vi "Compare-Results.vi"(10 "FFT {X}":csg[](array[numeric]), 11 "Array in":csg[](array[numeric])) -> (2 "Numeric":i32, 3 "Boolean":bool)   [LabVIEW 2015]
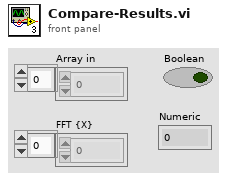
[diagram p1: front panel]
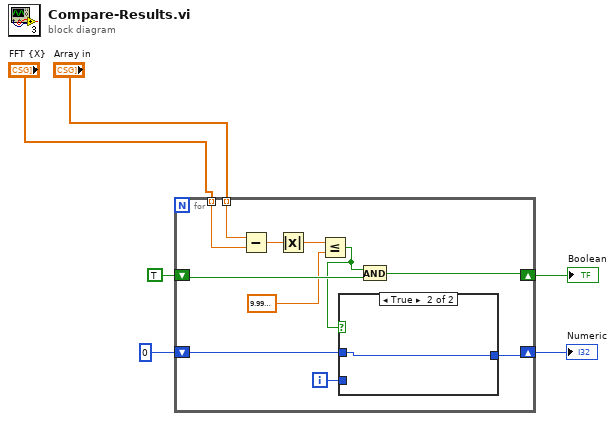
[diagram p0: block diagram]
diagram:
  n1 = for {
    shift-right: [w17] -> w2
    shift-left: TRUE -> [w16]
    tunnel: "FFT {X}" -> [w14] mode=indexing
    tunnel: "Array in" -> [w15] mode=indexing
    shift-right: [w8] -> w4
    shift-left: 0 -> [w7]
    i -> [w9]
    n2 = Subtract(x=w15, y=w14) -> (x-y=w13:csg)
    n3 = Absolute Value(x=w13) -> (abs(x)=w12:sgl)
    n4 = Less Or Equal?(x=w12, y=sgl 0.0001) -> (x <= y?=w10:bool)
    n5 = case shown="True" w10 {
      tunnel: w9 -> [w18 _]
      tunnel: [w18 w19] -> w8
      tunnel: w7 -> [_ w19]
      frame False {
      }
      frame True {
      }
    }
    n6 = And(x=w10, y=w16) -> (x .and. y?=w17:bool)
  }
  "Numeric" <- w4
  "Boolean" <- w2
